vi "JSON Flatten Configuration.vi"(8 "error in (no error)":errorcluster, 11 "configuration":T2={"plugins"=[{"core"={"name"="Plugin", "components"=[], "cycle timing"={"priority"=10000, "decimation"=1, "offset"=0}}, "component settings"=[], "threads"=[]}]}) -> (0 "error out":errorcluster, 2 "actual file version":T1, 3 "configuration json":string)   [LabVIEW 2019, in "DSF Core.lvlib" / "Configuration Session.lvclass"]
uses:
  Configuration Session.lvclass
  Typedefs/DSF Engine Framework Configuration.ctl
  Typedefs/DSF Engine Plugin Configuration.ctl
  Typedefs/Core Plugin Configuration.ctl
  Typedefs/DSF Timing Info.ctl
  Typedefs/DSF Settings Info.ctl
  Typedefs/DSF Engine Plugin Thread Configuration.ctl
  Typedefs/Core Thread Configuration.ctl
  Typedefs/DSF Engine Transfer Group Configuration.ctl
  Typedefs/Core Group Configuration.ctl
  Typedefs/DSF Direction.ctl
  Typedefs/DSF Timeout Behavior.ctl
  Typedefs/DSF Engine Transfer Configuration.ctl
  Typedefs/Core Transfer Configuration.ctl
  Typedefs/DSF Engine Channel Configuration.ctl
  Typedefs/Core Channel Configuration.ctl
  Typedefs/DSF Data Type.ctl
  Typedefs/DSF Version Info.ctl
  DSF Core.lvlib
  Configuration/Core/Channel/Channel Configuration.lvclass
  Configuration/Core/Transfer/Transfer Configuration.lvclass
  Configuration/Core/Group/Group Configuration.lvclass
  Configuration/Core/Thread/Thread Configuration.lvclass
  Configuration/Core/Plugin/Plugin Configuration.lvclass
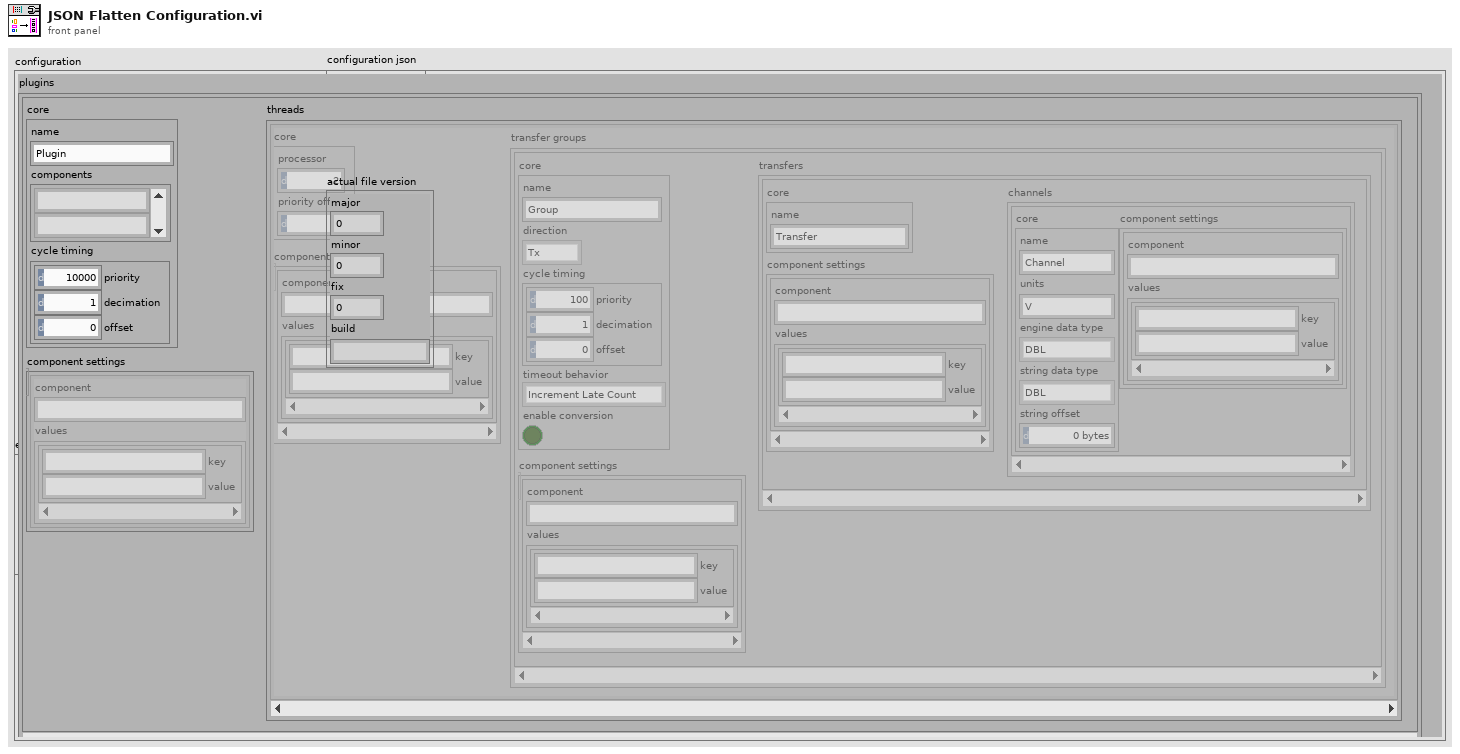
[diagram p1: front panel]
types:
  T1 = typedef "DSF Core.lvlib/DSF Version Info.ctl" = cluster{"major":u32, "minor":u32, "fix":u32, "build":string}
  T2 = typedef "DSF Core.lvlib/DSF Engine Framework Configuration.ctl" = cluster{"plugins":T3[]}
  T3 = typedef "DSF Core.lvlib/DSF Engine Plugin Configuration.ctl" = cluster{"core":T4, "component settings":T6[], "threads":T7[]}
  T4 = typedef "DSF Core.lvlib/Plugin Configuration.lvclass/Core Plugin Configuration.ctl" = cluster{"name":string, "components":string[], "cycle timing":T5}
  T5 = typedef "DSF Core.lvlib/DSF Timing Info.ctl" = cluster{"priority":u64, "decimation":u64, "offset":u64}
  T6 = typedef "DSF Core.lvlib/DSF Settings Info.ctl" = cluster{"component":string, "values":cluster{"key":string, "value":string}[]}
  T7 = typedef "DSF Core.lvlib/DSF Engine Plugin Thread Configuration.ctl" = cluster{"core":T8, "component settings":T6[], "transfer groups":T9[]}
  T8 = typedef "DSF Core.lvlib/Thread Configuration.lvclass/Core Thread Configuration.ctl" = cluster{"processor":i32, "priority offset":i16}
  T9 = typedef "DSF Core.lvlib/DSF Engine Transfer Group Configuration.ctl" = cluster{"core":T10, "component settings":T6[], "transfers":T13[]}
  T10 = typedef "DSF Core.lvlib/Group Configuration.lvclass/Core Group Configuration.ctl" = cluster{"name":string, "direction":T11, "cycle timing":T5, "timeout behavior":T12, "enable conversion":bool}
  T11 = typedef "DSF Core.lvlib/DSF Direction.ctl" = enum8{"Tx", "Rx"}
  T12 = typedef "DSF Core.lvlib/DSF Timeout Behavior.ctl" = enum8{"Increment Late Count", "Throw Error"}
  T13 = typedef "DSF Core.lvlib/DSF Engine Transfer Configuration.ctl" = cluster{"core":T14, "component settings":T6[], "channels":T15[]}
  T14 = typedef "DSF Core.lvlib/Transfer Configuration.lvclass/Core Transfer Configuration.ctl" = cluster{"name":string}
  T15 = typedef "DSF Core.lvlib/DSF Engine Channel Configuration.ctl" = cluster{"core":T16, "component settings":T6[]}
  T16 = typedef "DSF Core.lvlib/Channel Configuration.lvclass/Core Channel Configuration.ctl" = cluster{"name":string, "units":string, "engine data type":T17, "string data type":T17, "string offset":u64}
  T17 = typedef "DSF Core.lvlib/DSF Data Type.ctl" = enum8{"Bool", "SGL", "DBL", "I8", "I16", "I32", "I64", "U8", "U16", "U32", "U64"}
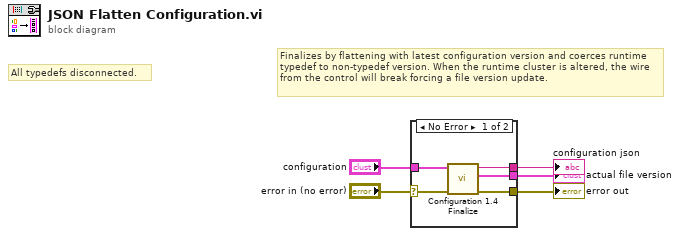
[diagram p0: block diagram]
diagram:
  # "Finalizes by flattening with latest configuration version and coerces runtime typedef to non-typedef version. When the runtime cluster is altered, the wire from the control will break forcing a file version update."
  # "All typedefs disconnected."
  n1 = case shown="No Error" "error in (no error)" {
    selector: "error in (no error)" -> [w9 w11]
    tunnel: [w6 w11] -> w5
    tunnel: [w8 _] -> w3
    tunnel: [w7 _] -> w2
    tunnel: "configuration" -> [w10 _]
    frame No Error {
      n2 = call "Configuration 1.4 Finalize.vi"("error in (no error)"=w9, "configuration 1.4"=w10) -> ("error out"=w6:errorcluster, "final file version"=w7:T1, "configuration json"=w8:string)  [unwired: 7 in]
    }
    frame Error {
    }
  }
  "configuration json" <- w3
  "error out" <- w5
  "actual file version" <- w2
